vi "Replace_Character.vi"(2 "Replace with":string, 3 "Input String":string, 4 "Search For":string) -> (0 "Matched Characters":string, 1 "Output string":string)   [LabVIEW 2020]
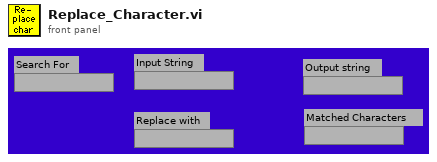
[diagram p1: front panel]
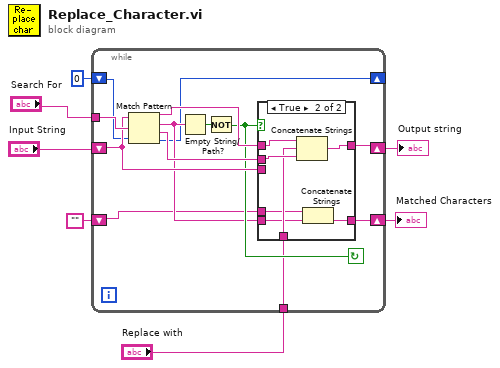
[diagram p0: block diagram]
diagram:
  n1 = while {
    shift-left: 0 ("offset past match") -> [w9]
    shift-right: [w8] -> _
    shift-left: "" -> [w11]
    shift-right: [w10] -> w2
    tunnel: "Replace with" -> [w13]
    shift-left: "Input String" -> [w17]
    shift-right: [w18] -> w6
    tunnel: "Search For" -> [w20]
    stop <- w14 continue-if-true
    n2 = Match Pattern(string=w17, regular expression=w20, offset (0)=w9) -> (before substring=w16:string, match substring=w12:string, after substring=w15:string, offset past match=w8:i32)
    n3 = Empty String/Path?(string/path=w12) -> (empty?=w19:bool)
    n4 = Not(x=w19) -> (.not. x?=w14:bool)
    n5 = case shown="True" w14 {
      tunnel: [w22 w28] -> w18
      tunnel: w17 -> [w22 _]
      tunnel: w16 -> [_ w29]
      tunnel: w15 -> [_ w27]
      tunnel: w13 -> [_ w26]
      tunnel: w12 -> [_ w25]
      tunnel: w11 -> [w21 w24]
      tunnel: [w21 w23] -> w10
      frame False {
      }
      frame True {
        n6 = Concatenate Strings(w29, w26, w27) -> (w28:string)
        n7 = Concatenate Strings(w24, w25) -> (w23:string)
      }
    }
  }
  "Output string" <- w6
  "Matched Characters" <- w2
